vi "Read Signal Generator.lvclass.vi"(11 "Switching Time in":refnum<class "Switching Time.lvclass">) -> (2 "Signal Generator.lvclass":refnum<class "Signal Generator.lvclass">, 3 "Switching Time out":refnum<class "Switching Time.lvclass">)   [LabVIEW 2020, in "Switching Time.lvclass"]
uses:
  Switching Time.lvclass
  Instruments/Signal Generator/Signal Generator.lvclass
  Switching Time.lvclass/Switching Time.ctl
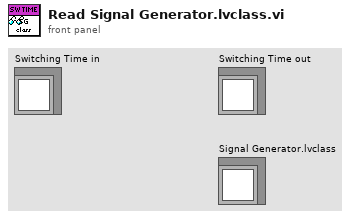
[diagram p1: front panel]
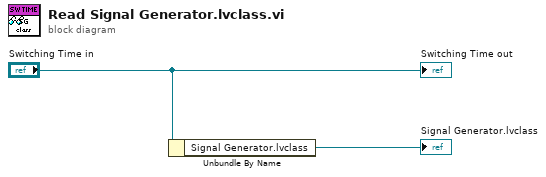
[diagram p0: block diagram]
diagram:
  n1 = Unbundle By Name("Switching Time in") -> ("Signal Generator.lvclass"=→"Signal Generator.lvclass":refnum<class "Signal Generator.lvclass">)
  "Switching Time out" <- "Switching Time in"
